vi "Wait until done.vi"(8 "error in (no error)":errorcluster, 10 "Event Registration":refnum<event-registration>, 11 "Execution API In":refnum<class "Execution API.lvclass">) -> (0 "error out":errorcluster, 2 "Output":string, 3 "Execution API Out":refnum<class "Execution API.lvclass">)   [LabVIEW 2020, in "Execution API.lvclass"]
doc: "Waits until all tests have been executed. The Result Events is obtained from the Register for Events.vi"
uses:
  Execution API.lvclass
  Core/Result/Result.ctl
  Core/Result/Status.ctl
  Core/Result/Type.ctl
  Execution API.lvclass/Execution API.ctl
  Core/Result/Result.lvlib
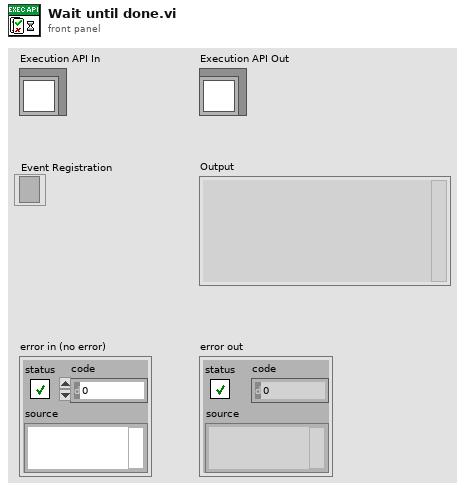
[diagram p1: front panel]
types:
  T1 = typedef "Result.lvlib/Status.ctl" = enum16{"", "Passed", "Failed", "Error", "Skipped", "Setup Error", "Broken", "Teardown Error"}
  T2 = typedef "Result.lvlib/Type.ctl" = enum16{"Test Case", "Test Suite", "Test Run", "Pass", "Fail", "Skip", "Pass if", "Fail if", "Pass if Error", "Fail if Error", "Pass if Equal", "Fail if Equal"}
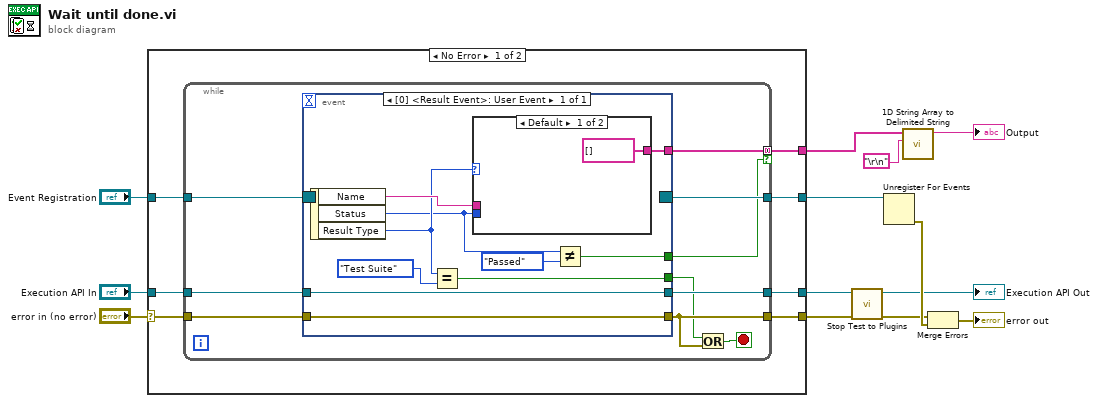
[diagram p0: block diagram]
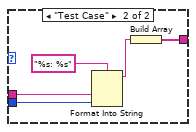
[diagram p2: hidden frame]
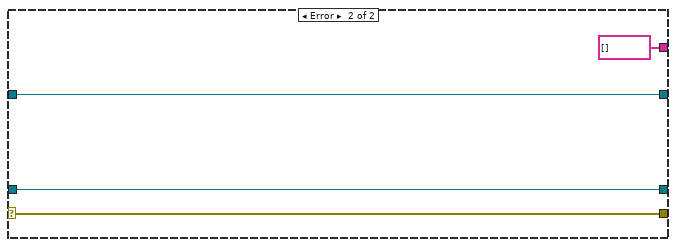
[diagram p3: hidden frame]
diagram:
  n1 = case shown="No Error" "error in (no error)" {
    selector: "error in (no error)" -> [w18 w50]
    tunnel: [w14 string[] []] -> w13
    tunnel: "Execution API In" -> [w20 w49]
    tunnel: [w19 w49] -> w2
    tunnel: [w17 w50] -> w9
    tunnel: [w16 w48] -> w4
    tunnel: "Event Registration" -> [w15 w48]
    frame No Error {
      n2 = while {
        tunnel: w15 -> [w30]
        tunnel: w18 -> [w27]
        tunnel: w20 -> [w28]
        tunnel: [w26] -> w19
        tunnel: [w25] -> w17
        tunnel: [w29] -> w16
        tunnel: [w22] -> w14 mode=concatenating if=w21
        stop <- w24 stop-if-true
        n3 = event shown="[0] <Result Event>: User Event" {
          selector: w30 -> [_]
          dyn-events: [_] -> w29
          timeout: _ -> [_]
          tunnel: w28 -> [w31]
          tunnel: w27 -> [w40]
          tunnel: [w31] -> w26
          tunnel: [w40] -> w25
          tunnel: [w38] -> w23
          tunnel: [w36] -> w22
          tunnel: [w32] -> w21
          event User Event {
            n4 = event-data() -> ("Name"=w37:string, "Status"=w34:T1, "Result Type"=w35:T2)  [unwired: 1 in]
            n5 = Equal?(x=w35, y=Type."Test Suite") -> (x = y?=w38:bool)
            n6 = case shown="Default" w35 {
              tunnel: w37 -> [_ w45]
              tunnel: w34 -> [_ w44]
              tunnel: [string[] [] w42] -> w36
              frame Default {
              }
              frame "Test Case" {
                n7 = Format Into String(format string="%s: %s", w45, w44) -> (resulting string=w43:string)  [unwired: 2 in, 1 out]
                n8 = Build Array(w43) -> (w42:string[])
              }
            }
            n9 = Not Equal?(x=w34, y=Status."Passed") -> (x != y?=w32:bool)
          }
        }
        n10 = Or(x=w23, y=w25) -> (x .or. y?=w24:bool)
      }
    }
    frame Error {
    }
  }
  n11 = call "Stop Test to Plugins.vi"("error in (no error)"=w9, "Execution API in"=w2) -> ("error out"=w3:errorcluster, "Execution API out"=→"Execution API Out":refnum<class "Execution API.lvclass">)  [unwired: 8 in]
  n12 = Unregister For Events(event registration refnum=w4) -> (error out=w6:errorcluster)  [unwired: 1 in]
  n13 = call <vilib>:"1D String Array to Delimited String.vi"("delimiter"="\r\n", "string array"=w13) -> ("delimited string"=→"Output":string)  [unwired: 9 in]
  n14 = Merge Errors(w3, w6) -> (→"error out":errorcluster)
